vi "Set All Column Params.vi"(8 "error in (no error)":errorcluster, 10 "ColumnSetup":T1[](array[typedef]) {"MinWidth" min=2 step=1; "AutoSizeMode" items=["None"=1, "ColumnHeader"=2, "AllCellsExceptHeader"=4, "AllCells"=6, "DisplayedCellsExceptHeader"=8, "DisplayedCells"=10, "Fill"=16]; "FillWeight" min=1 max=100}, 11 "DataTable in":refnum<class "DataTable.lvclass">) -> (0 "error out":errorcluster, 3 "DataTable out":refnum<class "DataTable.lvclass">)   [LabVIEW 2016, in "DataGrid.lvlib" / "DataTable.lvclass"]
uses:
  <userlib>/LabVIEWdotNetDataGrid/source/DataTable/DataTable.lvclass
  <userlib>/LabVIEWdotNetDataGrid/source/GridColumn/ColumnDefinition.ctl
  <userlib>/LabVIEWdotNetDataGrid/source/GridColumn/ColumnType.ctl
  <userlib>/LabVIEWdotNetDataGrid/source/DataTable/DataTable.lvclass/DataTable.ctl
  <userlib>/LabVIEWdotNetDataGrid/source/GridColumn/GridColumn.lvclass/GridColumn.ctl
  <userlib>/LabVIEWdotNetDataGrid/source/GridColumn/Write Name.vi
  <userlib>/LabVIEWdotNetDataGrid/source/GridColumn/Write datatype.vi
  <userlib>/LabVIEWdotNetDataGrid/source/GridColumn/Write Params.vi
  <userlib>/LabVIEWdotNetDataGrid/source/GridColumn/Write AutoSizeMode.vi
  <userlib>/LabVIEWdotNetDataGrid/source/GridColumn/Write Caption.vi
  <userlib>/LabVIEWdotNetDataGrid/source/GridColumn/Write Tooltip.vi
  <userlib>/LabVIEWdotNetDataGrid/source/GridColumn/Write ReadOnly.vi
  <userlib>/LabVIEWdotNetDataGrid/source/GridColumn/Write Visible.vi
  <userlib>/LabVIEWdotNetDataGrid/source/GridColumn/Write FillWeight.vi
  <userlib>/LabVIEWdotNetDataGrid/source/GridColumn/GridColumn.lvclass
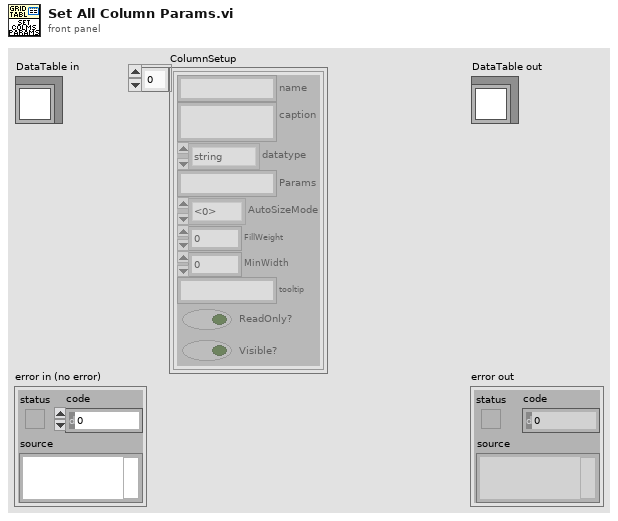
[diagram p1: front panel]
types:
  T1 = typedef "DataGrid.lvlib/GridColumn.lvclass/ColumnDefinition.ctl" = cluster{"name":string, "caption":string, "datatype":T2, "Params":string, "AutoSizeMode":i32, "FillWeight":sgl, "MinWidth":u32, "tooltip":string, "ReadOnly?":bool, "Visible?":bool}
  T2 = typedef "DataGrid.lvlib/GridColumn.lvclass/ColumnType.ctl" = enum16{"string", "image", "check", "numeric", "timestamp", "button", "combo", "link"}
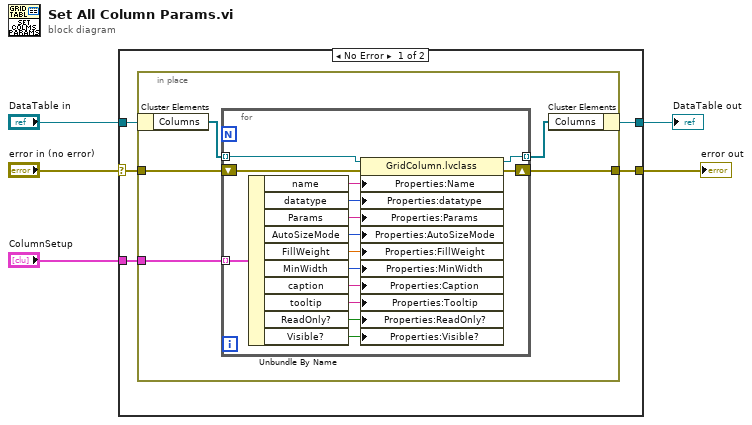
[diagram p0: block diagram]
diagram:
  n1 = case shown="No Error" "error in (no error)" {
    selector: "error in (no error)" -> [w9 w31]
    tunnel: [w8 w31] -> w4
    tunnel: [w6 w32] -> w2
    tunnel: "DataTable in" -> [w7 w32]
    tunnel: "ColumnSetup" -> [w10 _]
    frame No Error {
      n2 = in-place {
        in-place-border: w10 -> [w15]
        in-place-border: w9 -> [w14]
        in-place-border: [w13] -> w8
        n3 = in-place-cluster #1(w7) -> ("Columns"=w12:refnum<class "GridColumn.lvclass">[])
        n4 = for {
          tunnel: w15 -> [w20] mode=indexing
          shift-right: [w16] -> w13
          shift-left: w14 -> [w17]
          tunnel: [w18] -> w11 mode=indexing
          tunnel: w12 -> [w19] mode=indexing
          n5 = Unbundle By Name(w20) -> ("name"=w27:string, "datatype"=w26:T2, "Params"=w28:string, "AutoSizeMode"=w29:i32, "FillWeight"=w30:sgl, "MinWidth"=w25:u32, "caption"=w24:string, "tooltip"=w23:string, "ReadOnly?"=w22:bool, "Visible?"=w21:bool)
          n6 = property class="GridColumn.lvclass"(reference=w19, error in=w17, "Properties:Name"=w27, "Properties:datatype"=w26, "Properties:Params"=w28, "Properties:AutoSizeMode"=w29, "Properties:FillWeight"=w30, "Properties:MinWidth"=w25, "Properties:Caption"=w24, "Properties:Tooltip"=w23, "Properties:ReadOnly?"=w22, "Properties:Visible?"=w21) -> (reference out=w18:refnum<class "GridColumn.lvclass">, error out=w16:errorcluster)
        }
        n7 = in-place-cluster #1("Columns"=w11) -> (w6:refnum<class "DataTable.lvclass">)
      }
    }
    frame Error {
    }
  }
  "error out" <- w4
  "DataTable out" <- w2
